vi "setup Motor PWM LV.vi"(9 "motorFrequency":u16, 10 "motorEnables":u8, 11 "instance":i32) -> (3 "function return":u32)   [LabVIEW 2025, in "SADI_FW3.lvlib"]
doc: "SADI_API_Wrapper unsigned int setupMotorPWM_LV( int instance, uint8_t motorEnables, uint16_t motorFrequency );"
uses:
  SADI_FW3.lvlib
  SADI_FW3.dll
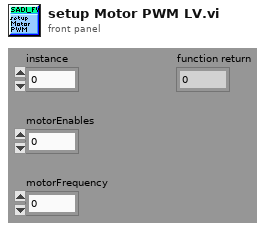
[diagram p1: front panel]
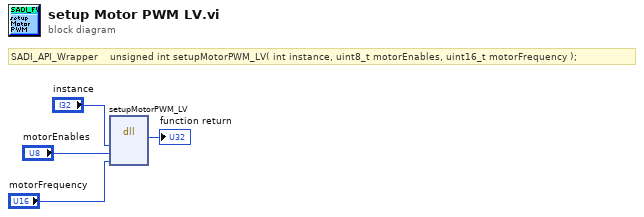
[diagram p0: block diagram]
diagram:
  # "SADI_API_Wrapper    unsigned int setupMotorPWM_LV( int instance, uint8_t motorEnables, uint16_t motorFrequency );"
  n1 = dll-call lib="C:/Users/noaht/School/Fall 2025/Controls Lab/Lab 3/EML4314c_FA25_framework_0/LVLib/SADI_FW3.*" fn="setupMotorPWM_LV"("instance"="instance", "motorEnables"="motorEnables", "motorFrequency"="motorFrequency") -> (→"function return":u32)  [unwired: 6 in, 2 out]
